vi "Export - Buffered Rx Packet.vi"(8 "error in (no error)":errorcluster, 11 "Device Item Ref in":T9 format="%.0x") -> (0 "error out":errorcluster, 3 "Rx Packet":T1 {"targetPriority" min=-2 max=16 step=1; "targetProcessor" min=-2 max=16 step=1; "Endianness" items=["big-endian"=0, "little-endian"=2]})   [LabVIEW 2016, in "UDP-Custom-Device System Explorer.lvlib"]
uses:
  UDP-Custom-Device System Explorer.lvlib
  <vilib>/NI Veristand/Custom Device API/Custom Device Item Ref.ctl
  Types/XML - New/ImpExp - Rx Packet Data.ctl
  <vilib>/NI Veristand/Custom Device API/Custom Device Item Info.ctl
  Shared/Types/Shared - Channel Data Type.ctl
  Shared/Types/Shared - Buffered.PacketInfo.ctl
  Shared/Types/Shared - Pointer Encoding.ctl
  Shared/Types/Shared - Receive Buffer Options.ctl
  Shared/Types/Shared - Transmit Buffer Options.ctl
  Shared/Types/Shared - New Data Options.ctl
  Shared/UDP-Custom-Device Shared.lvlib
  <vilib>/NI VeriStand/Custom Device API/Custom Device API.lvlib
  Property Accessors/Shared Packet Accessors.lvlib
  Property Accessors/Rx Packet Accessors.lvlib
  Property Accessors/Buffered Data Packet.lvlib
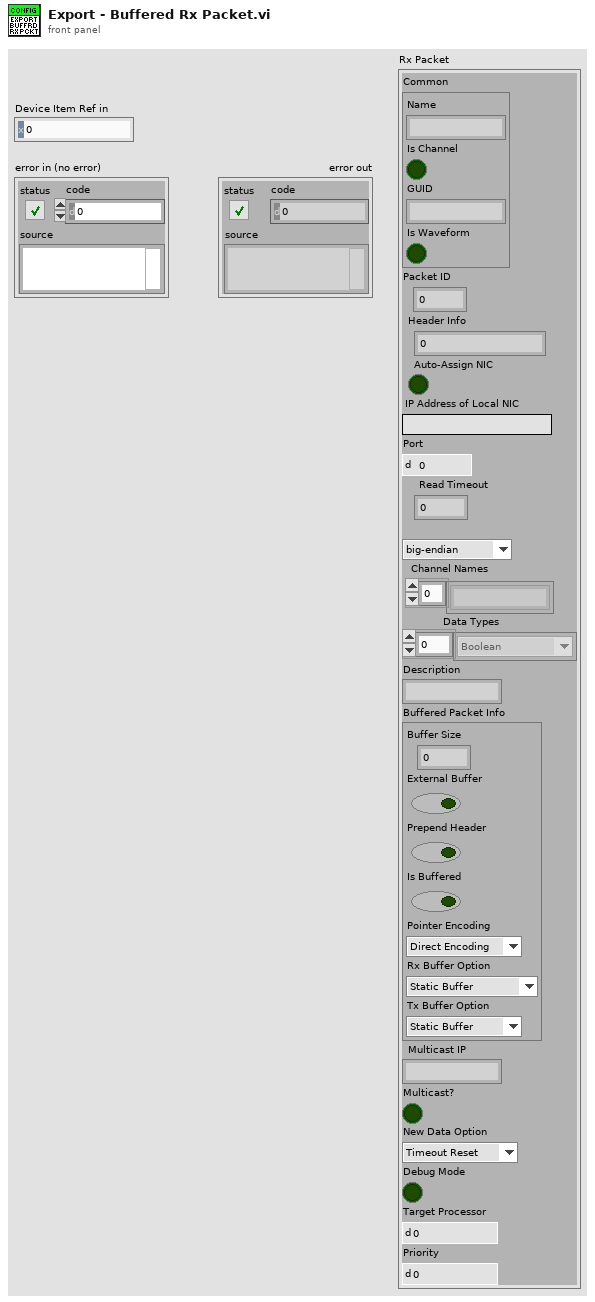
[diagram p1: front panel]
types:
  T1 = typedef "UDP-Custom-Device System Explorer.lvlib/ImpExp - Rx Packet Data.ctl" = cluster{"Common":T2, "Packet ID":i32, "Header Info":u32, "Auto-Assign NIC":bool, "IP Address of Local NIC":string, "Port":u16, "Read Timeout":i32, "Endianness":u16, "Channel Names":string[], "Data Types":T3[], "Description":string, "Buffered Packet Info":T4, "Multicast IP":string, "Multicast?":bool, "New Data Option":T8, "Debug Mode":bool, "targetProcessor":i8, "targetPriority":i16}
  T2 = typedef "Custom Device API.lvlib/Custom Device Item Info.ctl" = cluster{"Name":string, "Is Channel":bool, "GUID":string, "Is Waveform":bool}
  T3 = typedef "UDP-Custom-Device Shared.lvlib/Shared - Channel Data Type.ctl" = enum16{"Boolean", "Single", "Double", "I8", "I16", "I32", "I64", "U8", "U16", "U32", "U64"}
  T4 = typedef "UDP-Custom-Device Shared.lvlib/Shared - Buffered.PacketInfo.ctl" = cluster{"Buffer Size":i32, "External Buffer":bool, "Prepend Header":bool, "Is Buffered":bool, "Pointer Encoding":T5, "Rx Buffer Option":T6, "Tx Buffer Option":T7}
  T5 = typedef "UDP-Custom-Device Shared.lvlib/Shared - Pointer Encoding.ctl" = enum16{"Direct Encoding", "Conversion Encoding"}
  T6 = typedef "UDP-Custom-Device Shared.lvlib/Shared - Receive Buffer Options.ctl" = enum16{"Static Buffer", "Circular Buffer", "Circular Buffer + Size"}
  T7 = typedef "UDP-Custom-Device Shared.lvlib/Shared - Transmit Buffer Options.ctl" = enum16{"Static Buffer", "FIFO Buffer", "FIFO Buffer + Port"}
  T8 = typedef "UDP-Custom-Device Shared.lvlib/Shared - New Data Options.ctl" = enum16{"Timeout Reset", "Counter"}
  T9 = typedef "Custom Device API.lvlib/Custom Device Item Ref.ctl" = u64
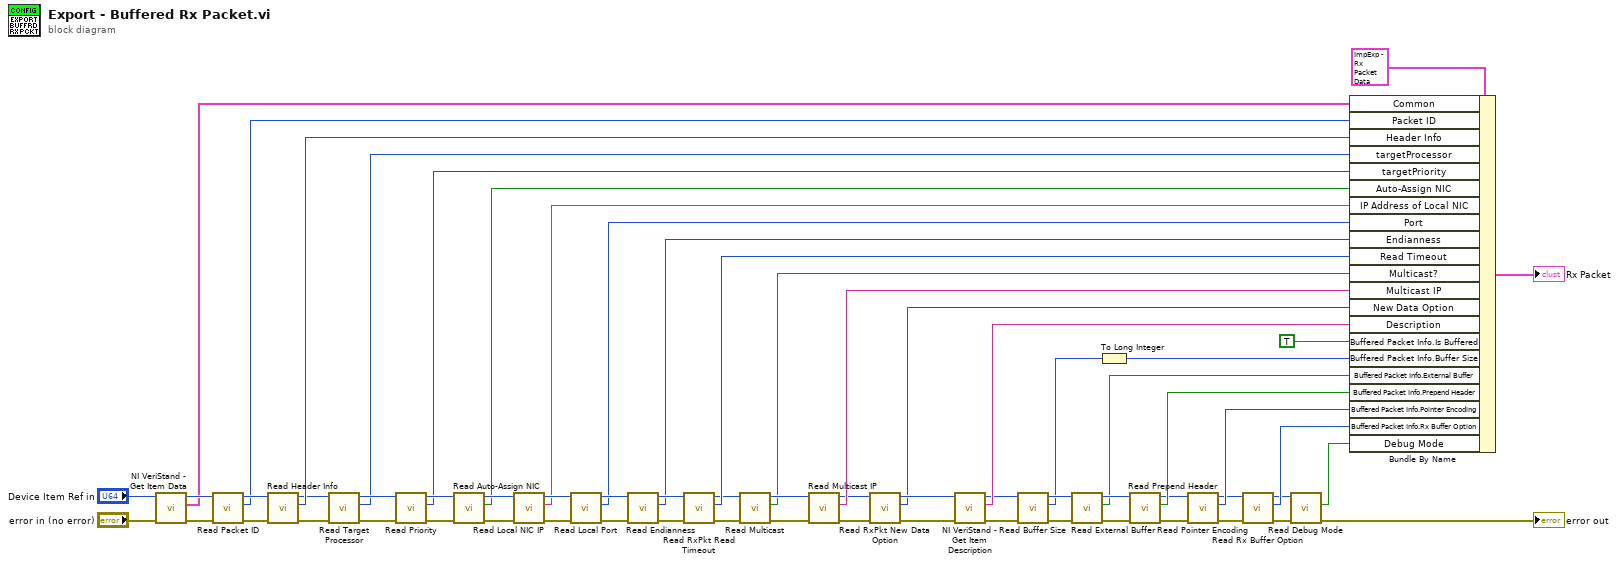
[diagram p0: block diagram]
diagram:
  n1 = call <vilib>:"NI VeriStand - Get Item Data.vi"("error in (no error)"="error in (no error)", "Item Ref in"="Device Item Ref in") -> ("error out"=w61:errorcluster, "Item Info"=w50:T2, "Item Ref out"=w54:T9)  [unwired: 6 in, 1 out]
  n2 = call "Read Packet ID.vi"("error in (no error)"=w61, "Node Ptr"=w54) -> ("error out"=w56:errorcluster, "Packet ID"=w49:i32, "Node Ptr out"=w55:T9)  [unwired: 7 in]
  n3 = call "Read Header Info.vi"("error in (no error)"=w56, "Node Ptr"=w55) -> ("error out"=w4:errorcluster, "Header Info"=w48:u32, "Node Ptr out"=w6:T9)  [unwired: 7 in]
  n4 = call "Read Target Processor.vi"("error in (no error)"=w4, "Node Ptr"=w6) -> ("error out"=w7:errorcluster, "targetProcessor"=w2:i8, "Node Ptr out"=w8:T9)  [unwired: 7 in]
  n5 = call "Read Priority.vi"("error in (no error)"=w7, "Node Ptr"=w8) -> ("error out"=w3:errorcluster, "targetPriority"=w1:i16, "Node Ptr out"=w5:T9)  [unwired: 7 in]
  n6 = call "Read Auto-Assign NIC.vi"("error in (no error)"=w3, "Node Ptr"=w5) -> ("error out"=w60:errorcluster, "Auto-Assign NIC"=w47:bool, "Node Ptr out"=w57:T9)  [unwired: 7 in]
  n7 = call "Read Local NIC IP.vi"("error in (no error)"=w60, "Node Ptr"=w57) -> ("error out"=w59:errorcluster, "IP Address of Local NIC"=w46:string, "Node Ptr out"=w58:T9)  [unwired: 7 in]
  n8 = call "Read Local Port.vi"("error in (no error)"=w59, "Node Ptr"=w58) -> ("error out"=w62:errorcluster, "Port"=w45:u16, "Node Ptr out"=w63:T9)  [unwired: 7 in]
  n9 = call "Read Endianness.vi"("error in (no error)"=w62, "Node Ptr"=w63) -> ("error out"=w64:errorcluster, "Endianness"=w44:u16, "Node Ptr out"=w65:T9)  [unwired: 7 in]
  n10 = call "Read RxPkt Read Timeout.vi"("error in (no error)"=w64, "Node Ptr"=w65) -> ("error out"=w24:errorcluster, "Read Timeout"=w43:i32, "Node Ptr out"=w25:T9)  [unwired: 7 in]
  n11 = call "Read Multicast.vi"("error in (no error)"=w24, "Node Ptr"=w25) -> ("error out"=w28:errorcluster, "Multicast"=w27:bool, "Node Ptr out"=w29:T9)  [unwired: 7 in]
  n12 = call "Read Multicast IP.vi"("error in (no error)"=w28, "Node Ptr"=w29) -> ("error out"=w18:errorcluster, "Multicast IP Address"=w26:string, "Node Ptr out"=w20:T9)  [unwired: 7 in]
  n13 = call "Read RxPkt New Data Option.vi"("error in (no error)"=w18, "Node Ptr"=w20) -> ("error out"=w17:errorcluster, "New Data Option"=w16:T8, "Node Ptr out"=w19:T9)  [unwired: 7 in]
  n14 = call <vilib>:"NI VeriStand - Get Item Description.vi"("error in (no error)"=w17, "Item Ref in"=w19) -> ("error out"=w35:errorcluster, "Description"=w42:string, "Item Ref out"=w40:T9)  [unwired: 6 in, 1 out]
  n15 = call "Read Buffer Size.vi"("error in (no error)"=w35, "Node Ptr"=w40) -> ("error out"=w37:errorcluster, "Buffer Size"=w34:u32, "Node Ptr out"=w39:T9)  [unwired: 7 in]
  n16 = call "Read External Buffer.vi"("error in (no error)"=w37, "Node Ptr"=w39) -> ("error out"=w36:errorcluster, "External Buffer"=w33:bool, "Node Ptr out"=w38:T9)  [unwired: 7 in]
  n17 = To Long Integer(number=w34) -> (32bit integer=w30:i32)
  n18 = call "Read Prepend Header.vi"("error in (no error)"=w36, "Node Ptr"=w38) -> ("error out"=w22:errorcluster, "Prepend Header"=w32:bool, "Node Ptr out"=w23:T9)  [unwired: 7 in]
  n19 = call "Read Pointer Encoding.vi"("error in (no error)"=w22, "Node Ptr"=w23) -> ("error out"=w14:errorcluster, "Pointer Encoding"=w21:T5, "Node Ptr out"=w15:T9)  [unwired: 7 in]
  n20 = call "Read Rx Buffer Option.vi"("error in (no error)"=w14, "Node Ptr"=w15) -> ("error out"=w11:errorcluster, "Buffer Option"=w13:T6, "Node Ptr out"=w12:T9)  [unwired: 7 in]
  n21 = call "Read Debug Mode.vi"("error in (no error)"=w11, "Node Ptr"=w12) -> ("error out"=→"error out":errorcluster, "Debug Mode"=w9:bool)  [unwired: 7 in, 1 out]
  n22 = Bundle By Name(cluster=T1 {"Common"={"Name"="", "Is Channel"=FALSE, "GUID"="", "Is Waveform"=FALSE}, "Packet ID"=0, "Header Info"=0, "Auto-Assign NIC"=FALSE, "IP Address of Local NIC"="", "Port"=0, "Read Timeout"=0, "Endianness"=0, "Channel Names"=[], "Data Types"=[], "Description"="", "Buffered Packet Info"={"Buffer Size"=0, "External Buffer"=FALSE, "Prepend Header"=FALSE, "Is Buffered"=FALSE, "Pointer Encoding"=enum."Direct Encoding", "Rx Buffer Option"=enum."Static Buffer", "Tx Buffer Option"=enum."Static Buffer"}, "Multicast IP"="", "Multicast?"=FALSE, "New Data Option"=enum."Timeout Reset", "Debug Mode"=FALSE, "targetProcessor"=0, "targetPriority"=0} ("Rx Packet"), "Common"=w50, "Packet ID"=w49, "Header Info"=w48, "targetProcessor"=w2, "targetPriority"=w1, "Auto-Assign NIC"=w47, "IP Address of Local NIC"=w46, "Port"=w45, "Endianness"=w44, "Read Timeout"=w43, "Multicast?"=w27, "Multicast IP"=w26, "New Data Option"=w16, "Description"=w42, "Buffered Packet Info.Is Buffered"=TRUE, "Buffered Packet Info.Buffer Size"=w30, "Buffered Packet Info.External Buffer"=w33, "Buffered Packet Info.Prepend Header"=w32, "Buffered Packet Info.Pointer Encoding"=w21, "Buffered Packet Info.Rx Buffer Option"=w13, "Debug Mode"=w9) -> (→"Rx Packet":T1)
